vi "SLSC Calibrate UEGO.vi"(7 "settings.SLSC":T2={"SPI PHY Settings"={"Divide Value"=20, "Transfer Length (bits)"=32, "CS Asserted Polarity"=FALSE, "Clock Polarity (CPOL)"=FALSE, "Clock Phase (CPHA)"=FALSE, "Lengthen MISO Setup"=FALSE, "Direction Change Bit"=0, "MOSI Starts as Output"=FALSE, "Tristatable MOSI"=FALSE}, "Sample Rate (S/s)"=10000} {"SPI PHY Settings"."Direction Change Bit" max=64 step=1; "SPI PHY Settings"."Transfer Length (bits)" min=1 max=64 step=1}, 8 "Calibrate?":refnum<k21>="Calibration?", 9 "CS Bits":T6={"CS Bit 1"="Connector0/DIO0", "CS Bit 2"="Connector0/DIO0", "CS Bit 3"="Connector0/DIO0", "CS Bit 4"="Connector0/DIO0"}, 10 "SPI DIO Lines":T4={"SCLK"="Port0/DIO3", "MISO"="Port0/DIO3", "MOSI"="Port0/DIO3", "CS 0"="Port0/DIO3", "CS 1"="Port0/DIO4", "CS 2"="Port0/DIO4", "CS 3"="Port0/DIO1", "CS 4"="Port0/DIO4", "CS 5"="Port0/DIO4"}, 11 "slsc.calibration":T5) -> (3 "Complete?":T1)   [LabVIEW 2014, in "SLSC FPGA Toolkit.lvlib"]
uses:
  SLSC FPGA Toolkit.lvlib
  Source/Shared/SPI Utility/CS Bits.ctl
  SLSC UEGO Calibration.ctl
  <vilib>/SPI API/SPIAPI/DIO/SPI Digital IO Lines.ctl
  SLSC FPGA Inputs.ctl
  <userlib>/_NI SPI IP/FPGA/Controllers/Public/Transfer Settings.ctl
  SLSC Calibration Complete.ctl
  SLSC UEGO Calibration States.ctl
  <vilib>/Platform/TimedLoop/XDataNode/timing_clust.ctl
  <vilib>/Platform/TimedLoop/XDataNode/nitl_modes.ctl
  <vilib>/Platform/TimedLoop/XDataNode/wakeup.ctl
  <vilib>/rvi/Emulation/niFpgaSctlEmulationGetInTimedLoop.vi
  <vilib>/rvi/Emulation/niFpgaProcessEmulError.vi
  <vilib>/rvi/Emulation/niFpgaEmulationReportErrorSimple.vi
  <vilib>/rvi/Emulation/niFpgaGetClockAttributes.vi
  <vilib>/rvi/Emulation/niFpgaCriticalErrorInLSC.vi
  <vilib>/rvi/DataTransferAndStorage/Container/Common/niFpgaContainerExecOnDevCompGetState.vi
  <vilib>/rvi/Emulation/niFpgaEmulationIsFPGAContextNoSignature.vi
  <vilib>/rvi/DataTransferAndStorage/Container/Common/niFpgaContainerGetUniqueNameForEmu.vi
  <vilib>/rvi/Memory/Memory_Emulation/niFpgaMemoryEmulationCacheClearOnFirstRun.vi
  <vilib>/rvi/Memory/Memory_Emulation/nirvimemoryEmulationManagerCache_MakeExclusive.vi
  <vilib>/rvi/Memory/Memory_Emulation/niFpgaMemoryEmulationValidateCache.vi
  <vilib>/rvi/Memory/Memory_Emulation/nirvimemoryEmulationManagerCache_InsertValue.vi
  <vilib>/Utility/error.llb/Clear Errors.vi
  <vilib>/rvi/Memory/Memory_Emulation/nirvimemoryEmulationManagerCache_ReleaseExclusive.vi
  <vilib>/rvi/Memory/Memory_Emulation/nirvimemoryEmulationManagerCache_GetValue.vi
  <vilib>/rvi/Memory/Memory_Emulation/nirvimemoryEmulationManagerCache_SetValue.vi
  <vilib>/rvi/eio/common/nirviEmuTemplateMethod_errors.vi
  <vilib>/Platform/TimedLoop/XDataNode/XDataNode.xnode
  <vilib>/rvi/DataTransferAndStorage/Container/XNode/niFpgaContainer.xnode
  <vilib>/rvi/DataTransferAndStorage/Register/Emulation/niFpgaRegisterEmulationRefIn.vi
  <vilib>/eio/EIONode/EIONode.xnode
  <vilib>/Platform/TimedLoop/XDataNode/XDNodeRunTimeDep.lvlib
  Source/Shared/SLSC configuration Shared.lvlib
  <userlib>/_NI SPI IP/FPGA/Controllers/NI SPI IP FPGA.lvlib
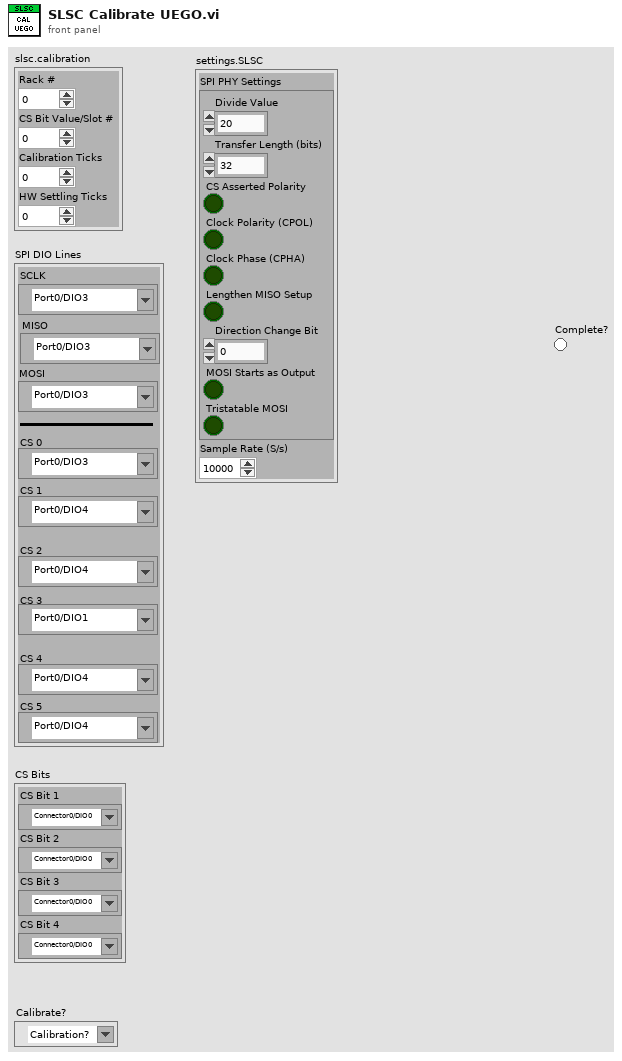
[diagram p1: front panel]
types:
  T1 = typedef "SLSC FPGA Toolkit.lvlib/SLSC Calibration Complete.ctl" = bool
  T2 = typedef "SLSC FPGA Toolkit.lvlib/SLSC FPGA Inputs.ctl" = cluster{"SPI PHY Settings":T3, "Sample Rate (S/s)":u32}
  T3 = typedef "NI SPI IP FPGA.lvlib/Transfer Settings.ctl" = cluster{"Divide Value":u8, "Transfer Length (bits)":u8, "CS Asserted Polarity":bool, "Clock Polarity (CPOL)":bool, "Clock Phase (CPHA)":bool, "Lengthen MISO Setup":bool, "Direction Change Bit":u8, "MOSI Starts as Output":bool, "Tristatable MOSI":bool}
  T4 = typedef "SPI Digital IO Lines.ctl" = cluster{"SCLK":refnum<k21>, "MISO":refnum<k21>, "MOSI":refnum<k21>, "CS 0":refnum<k21>, "CS 1":refnum<k21>, "CS 2":refnum<k21>, "CS 3":refnum<k21>, "CS 4":refnum<k21>, "CS 5":refnum<k21>}
  T5 = typedef "SLSC FPGA Toolkit.lvlib/SLSC UEGO Calibration.ctl" = cluster{"Rack #":u8, "CS Bit Value/Slot #":u8, "Calibration Ticks":u32, "HW Settling Ticks":u32}
  T6 = typedef "SLSC configuration Shared.lvlib/CS Bits.ctl" = cluster{"CS Bit 1":refnum<k21>, "CS Bit 2":refnum<k21>, "CS Bit 3":refnum<k21>, "CS Bit 4":refnum<k21>}
  T7 = typedef "SLSC FPGA Toolkit.lvlib/SLSC UEGO Calibration States.ctl" = enum16{"Initialize", "Assert CS", "Starts Calibration", "Stops Calibration", "Deassert CS", "Reset CS Bits"}
  T8 = typedef "XDNodeRunTimeDep.lvlib/timing_clust.ctl" = cluster{"Expected End [f-1]":u64, "Actual End [f-1]":u64, "Finished Late? [f-1]":bool, "Expected End [i-1]":u64, "Actual End [i-1]":u64, "Finished Late? [i-1]":bool, "Expected Start [i]":u64, "Actual Start [i]":u64, "Expected Start [f]":u64, "Actual Start [f]":u64, "Source Name":string, "Structure Name":string, "Period":i64, "Deadline":i64, "Offset":i64, "Start":i64, "Priority":i32, "Timeout":i32, "Mode":T9, "Wakeup Reason":T10, "Error":errorcluster, "Source Type":string, "Secondary Source Type":string, "Global End Time":u64, "Global Start Time":u64, "Frame Duration":u64, "Iteration Duration":u64, "Assigned CPU":i32, "I/O Scan Engine Mode":u32}
  T9 = typedef "XDNodeRunTimeDep.lvlib/nitl_modes.ctl" = enum32{"No Change", "Process missed periods, maintain original phase", "Discard missed periods, maintain original phase", "Process missed periods, ignore original phase", "Discard missed periods, ignore original phase"}
  T10 = typedef "XDNodeRunTimeDep.lvlib/wakeup.ctl" = enum32{"Normal", "Aborted", "Asynchronous wakeup", "Timing source error", "Timed loop error", "Timeout"}
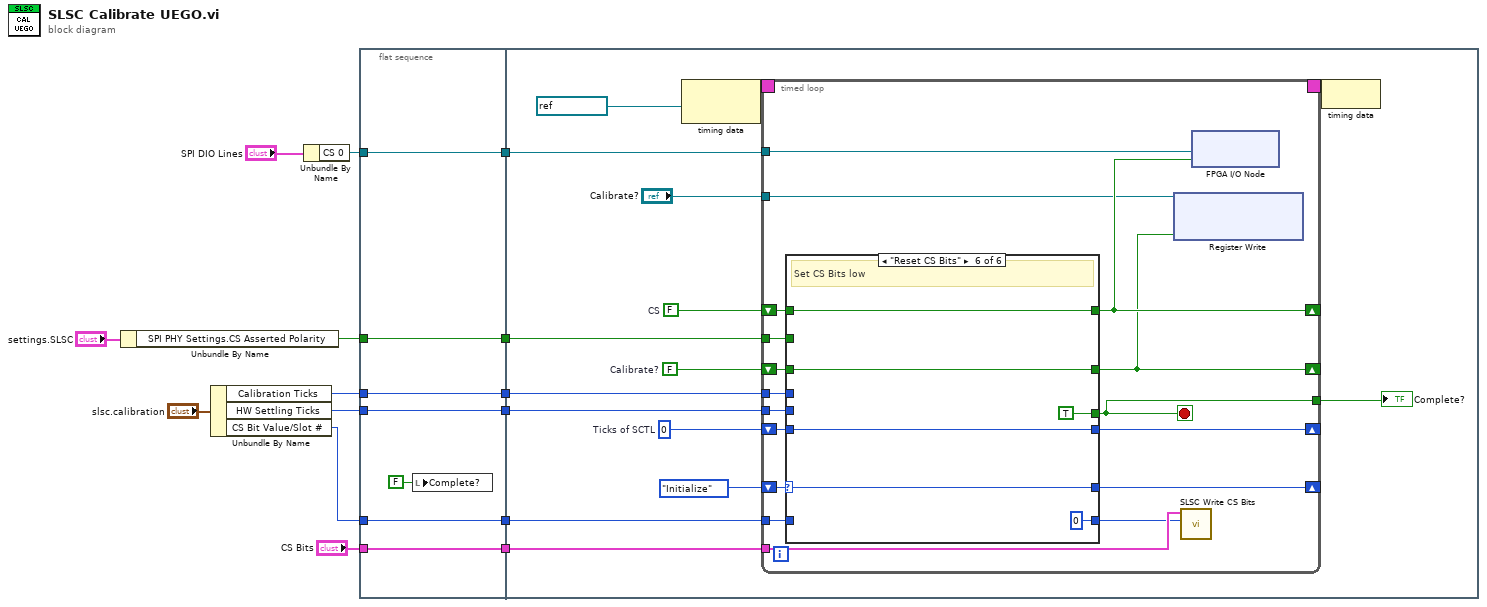
[diagram p0: block diagram]
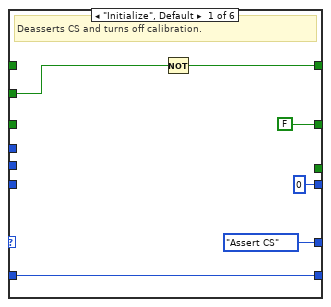
[diagram p2: hidden frame]
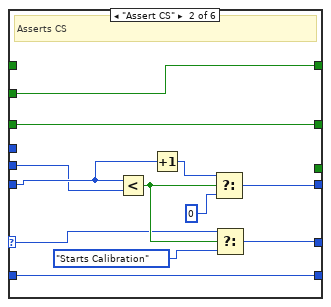
[diagram p3: hidden frame]
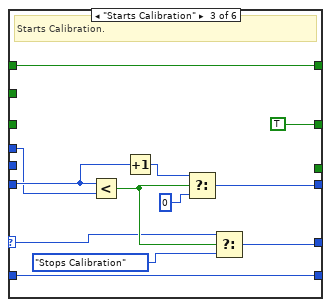
[diagram p4: hidden frame]
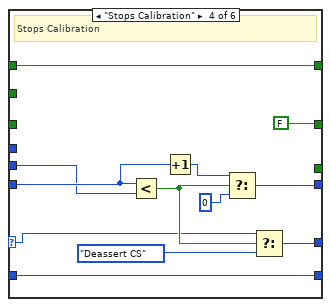
[diagram p5: hidden frame]
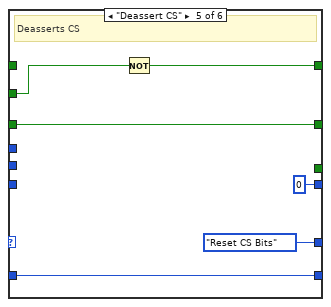
[diagram p6: hidden frame]
diagram:
  n1 = Unbundle By Name("settings.SLSC") -> ("SPI PHY Settings.CS Asserted Polarity"=w12:bool)
  n2 = Unbundle By Name("slsc.calibration") -> ("Calibration Ticks"=w9:u32, "HW Settling Ticks"=w8:u32, "CS Bit Value/Slot #"=w10:u8)
  n3 = Unbundle By Name("SPI DIO Lines") -> ("CS 0"=w14:refnum<k21>)
  n4 = flat-sequence {
    tunnel: w8 -> [w18]
    tunnel: w9 -> [w19]
    tunnel: w10 -> [w20]
    tunnel: w12 -> [w21]
    tunnel: w14 -> [w22]
    tunnel: [w22] -> w7
    tunnel: [w21] -> w6
    tunnel: [w20] -> w5
    tunnel: [w19] -> w4
    tunnel: [w18] -> w3
    tunnel: "CS Bits" -> [w16]
    tunnel: [w16] -> w1
    tunnel: w7 -> [w33]
    tunnel: w6 -> [w32]
    tunnel: w5 -> [w24]
    tunnel: w4 -> [w28]
    tunnel: w3 -> [w27]
    tunnel: w1 -> [w23]
    frame #0 {
      n5 = local write "Complete?"(T1 FALSE ("Complete?")) -> ()
    }
    frame #1 {
      w26 = FALSE  # Calibrate?
      w29 = u32 0  # Ticks of SCTL
      w31 = FALSE  # CS
      n6 = node-c288(refnum<k21> "120MHz" ("Source Name")) -> (w37:T8)
      n7 = timed-loop {
        shift-right: [w52] -> _
        shift-left: SLSC_UEGO_Calibration_States."Initialize" -> [w54]
        tunnel: w33 -> [w50]
        tunnel: w32 -> [w53]
        tunnel: "Calibrate?" -> [w43]
        tunnel: [w51] -> w25
        shift-right: [w49] -> _
        shift-left: w31 -> [w48]
        timing: w37 -> [_]
        timing-out: [_] -> w36
        shift-right: [w44] -> _
        shift-left: w29 -> [w47]
        tunnel: w28 -> [w46]
        tunnel: w27 -> [w45]
        shift-right: [w42] -> _
        shift-left: w26 -> [w41]
        tunnel: w24 -> [w40]
        tunnel: w23 -> [w39]
        stop <- w51 stop-if-true
        n8 = case shown="\"Reset CS Bits\"" w54 {
          selector: w54 -> [_ w65 w78 w90 _ w104]
          tunnel: [_ _ _ _ _ TRUE] -> w51
          tunnel: w53 -> [w60 w72 _ _ w102 _]
          tunnel: [SLSC_UEGO_Calibration_States."Assert CS" w64 w77 w89 SLSC_UEGO_Calibration_States."Reset CS Bits" w104] -> w52
          tunnel: [w59 w72 w84 w96 w101 w108] -> w49
          tunnel: w48 -> [_ _ w84 w96 _ w108]
          tunnel: w47 -> [_ w71 w80 w92 _ w105]
          tunnel: w46 -> [_ _ w76 _ _ _]
          tunnel: w45 -> [_ w67 _ w91 _ _]
          tunnel: [u32 0 ("f") w68 w79 w88 u32 0 ("f") w105] -> w44
          tunnel: [FALSE ("Calibrate?") w63 TRUE ("Calibrate?") FALSE ("Calibrate?") w99 w107] -> w42
          tunnel: w41 -> [_ w63 _ _ w99 w107]
          tunnel: w40 -> [w56 w62 w74 w86 w98 _]
          tunnel: [w56 w62 w74 w86 w98 u8 0 ("CS Bit Value/Slot #")] -> w38
          frame "Initialize", Default {
            # "Deasserts CS and turns off calibration."
            n9 = Not(x=w60) -> (.not. x?=w59:bool)
          }
          frame "Assert CS" {
            # "Asserts CS"
            n10 = Less?(x=w71, y=w67) -> (x < y?=w66:bool)
            n11 = Increment(x=w71) -> (x+1=w70:u32)
            n12 = Select(t=w70, s=w66, f=u16 0) -> (s? t:f=w68:u32)
            n13 = Select(t=w65, s=w66, f=SLSC_UEGO_Calibration_States."Starts Calibration") -> (s? t:f=w64:T7)
          }
          frame "Starts Calibration" {
            # "Starts Calibration."
            n14 = Less?(x=w80, y=w76) -> (x < y?=w81:bool)
            n15 = Increment(x=w80) -> (x+1=w83:u32)
            n16 = Select(t=w83, s=w81, f=u16 0) -> (s? t:f=w79:u32)
            n17 = Select(t=w78, s=w81, f=SLSC_UEGO_Calibration_States."Stops Calibration") -> (s? t:f=w77:T7)
          }
          frame "Stops Calibration" {
            # "Stops Calibration"
            n18 = Less?(x=w92, y=w91) -> (x < y?=w93:bool)
            n19 = Increment(x=w92) -> (x+1=w95:u32)
            n20 = Select(t=w95, s=w93, f=u16 0) -> (s? t:f=w88:u32)
            n21 = Select(t=w90, s=w93, f=SLSC_UEGO_Calibration_States."Deassert CS") -> (s? t:f=w89:T7)
          }
          frame "Deassert CS" {
            # "Deasserts CS"
            n22 = Not(x=w102) -> (.not. x?=w101:bool)
          }
          frame "Reset CS Bits" {
            # "Set CS Bits low"
          }
        }
        n23 = xnode ("Register Write")("Data"=w42, "Register In"=w43) -> ()  [unwired: 1 out]
        n24 = call "SLSC Write CS Bits.vi"("CS Bit Value/Slot #"=w38, "CS Bits"=w39) -> ()  [unwired: 10 in]
        n25 = xnode "FPGA I/O Node"("I/O Item"=w49, "FPGA I/O In"=w50) -> ()  [unwired: 1 out]
      }
      "Complete?" <- w25
      n26 = node-c288(w36) -> ()
    }
  }
